vi "AddArmpressureAndSave.vi"(8 "error in":errorcluster, 10 "Side(Left/Right)":string, 11 "data":T1) -> (0 "error out":errorcluster)   [LabVIEW 2013, in "main.lvlib"]
uses:
  main.lvlib
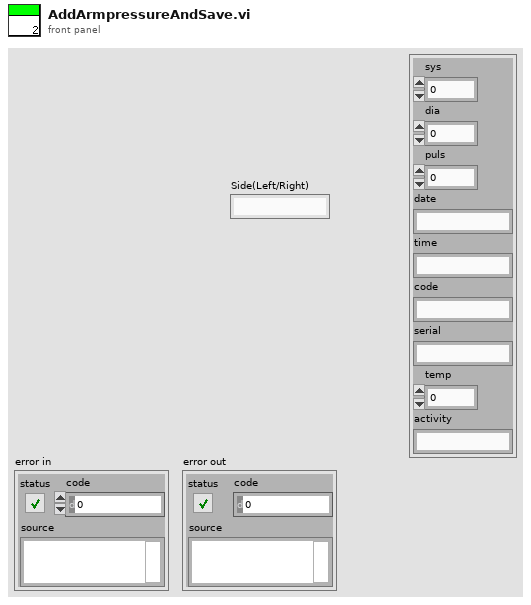
[diagram p1: front panel]
types:
  T1 = cluster{"sys":dbl, "dia":dbl, "puls":dbl, "date":string, "time":string, "code":string, "serial":string, "temp":dbl, "activity":string}
  T2 = typedef "main.lvlib/date_specific_info.ctl" = cluster{"profile":cluster{"id":string, "name":string, "operator":string, "doctor":string, "comment":string}, "hospital":cluster{"name":string, "department":string, "address":string}, "palpation":cluster{"right":string, "left":string}, "Armpressure Right":cluster{"sys":dbl, "dia":dbl, "puls":dbl, "date":string, "time":string, "code":string, "serial":string, "temp":dbl, "activity":string}[], "Armpressure Left":cluster{"sys":dbl, "dia":dbl, "puls":dbl, "date":string, "time":string, "code":string, "serial":string, "temp":dbl, "activity":string}[]}
  T3 = cluster{"sys":dbl, "dia":dbl, "puls":dbl, "date":string, "time":string, "code":string, "serial":string, "temp":dbl, "activity":string}[]
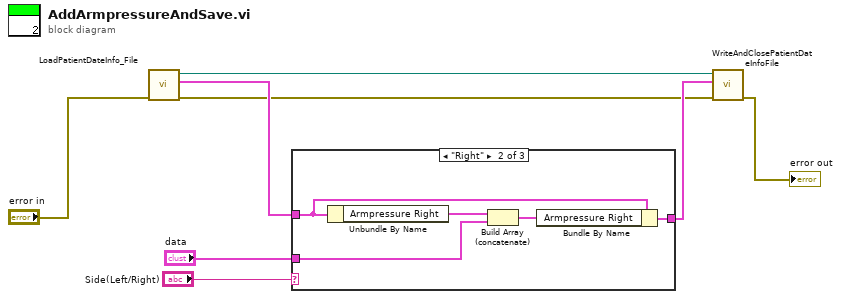
[diagram p0: block diagram]
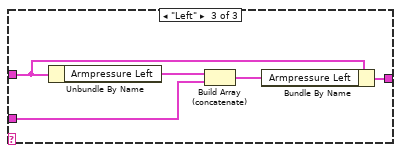
[diagram p3: hidden frame]
diagram:
  n1 = call "LoadPatientDateInfo_File.vi"("error in (no error)"="error in") -> ("error out"=w3:errorcluster, "date_specific_info"=w4:T2, "path"=w2:path)  [unwired: 8 in]
  n2 = case shown="\"Right\"" "Side(Left/Right)" {
    tunnel: [w9 w10 w19] -> w8
    tunnel: "data" -> [_ w12 w16]
    tunnel: w4 -> [w9 w11 w15]
    frame "False", Default {
    }
    frame "Right" {
      n3 = Unbundle By Name(w11) -> ("Armpressure Right"=w14:T3)
      n4 = Build Array (concatenate)(w14, w12) -> (w13:T3)
      n5 = Bundle By Name(cluster=w11, "Armpressure Right"=w13) -> (w10:T2)
    }
    frame "Left" {
      n6 = Unbundle By Name(w15) -> ("Armpressure Left"=w18:T3)
      n7 = Build Array (concatenate)(w18, w16) -> (w17:T3)
      n8 = Bundle By Name(cluster=w15, "Armpressure Left"=w17) -> (w19:T2)
    }
  }
  n9 = call "WriteAndClosePatientDateInfoFile.vi"("error in (no error)"=w3, "date_specific_info"=w8, "file path (use dialog)"=w2) -> ("error out"=→"error out":errorcluster)  [unwired: 8 in]
